vi "Poke-n-probe.vi"(6 "Tries":i32=150, 7 "Goal":T1, 8 "error in":errorcluster, 9 "Speed":dbl=15.0, 10 "Zone":dbl=5.0, 11 "Location":string="Base") -> (0 "error out":errorcluster, 1 "Speed Out":dbl, 2 "Success":bool, 3 "Location Out":string="Base", 5 "Pose":T1)   [LabVIEW 2013]
uses:
  ROS/Code/Console/Servers/ServerSubs/(nist) Arm Globals.vi
panel:
  in  "Tolerance":dbl
  out "Overload":dbl
  out "Try":i32
  in  "stop":bool
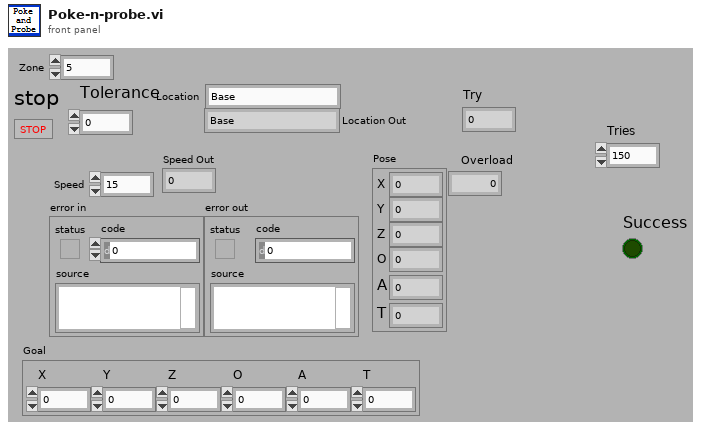
[diagram p1: front panel]
types:
  T1 = cluster{"X":dbl, "Y":dbl, "Z":dbl, "O":dbl, "A":dbl, "T":dbl}
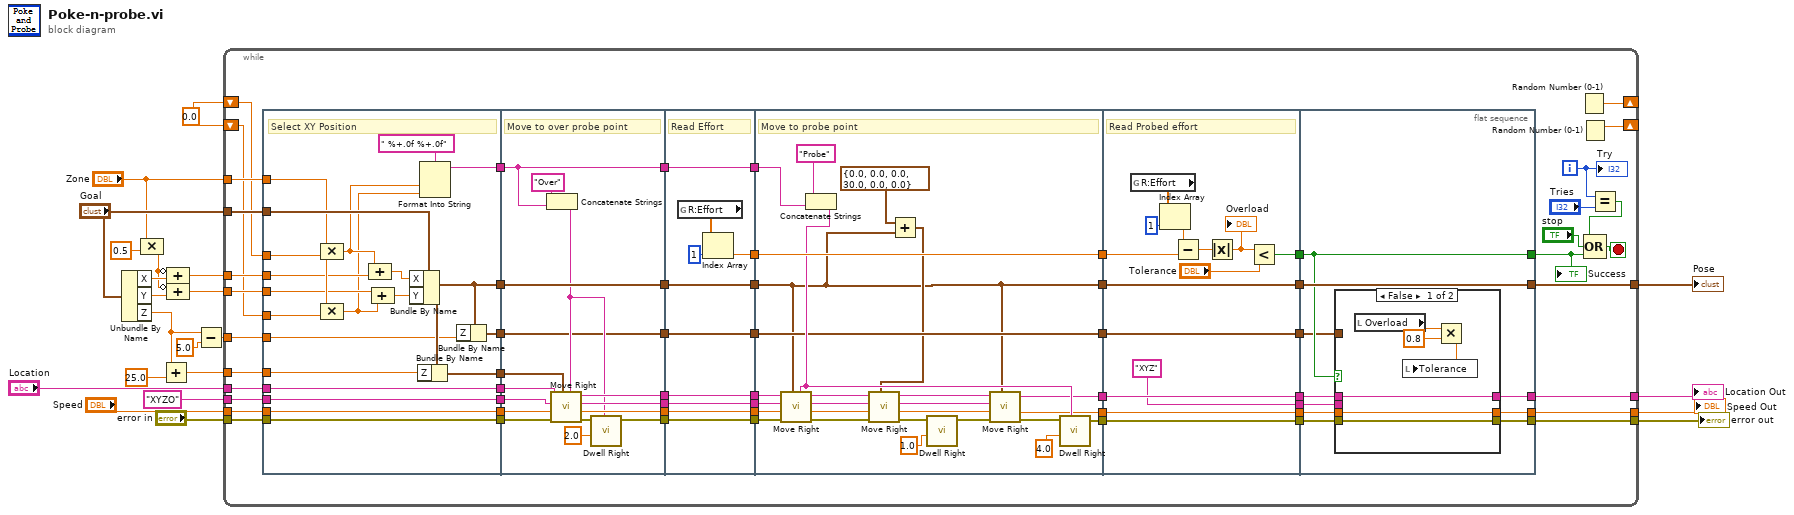
[diagram p0: block diagram]
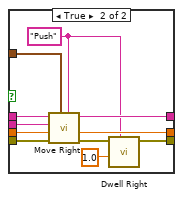
[diagram p2: hidden frame]
diagram:
  w1 = 0.0
  n1 = Unbundle By Name("Goal") -> ("X"=w15:dbl, "Y"=w14:dbl, "Z"=w4:dbl)
  n2 = Compound Arithmetic op=MULTIPLY("Zone", 0.5 ("value")) -> (w12:dbl)
  n3 = Add(x=w4, y=25.0 ("x")) -> (x+y=w17:dbl)
  n4 = Compound Arithmetic op=ADD(invert w12, w15) -> (w9:dbl)
  n5 = Compound Arithmetic op=ADD(invert w12, w14) -> (w10:dbl)
  n6 = Subtract(x=w4, y=5.0) -> (x-y=w2:dbl)
  n7 = while {
    tunnel: "error in" -> [w64]
    tunnel: "Location" -> [w63]
    tunnel: "XYZO" ("Mask") -> [w62]
    tunnel: "Speed" -> [w61]
    tunnel: w17 -> [w60]
    tunnel: "Goal" -> [w59]
    tunnel: "Zone" -> [w58]
    tunnel: w10 -> [w57]
    tunnel: w9 -> [w56]
    tunnel: [w54] -> w8
    tunnel: [w53] -> w5
    tunnel: [w51] -> w7
    tunnel: [w50] -> w6
    tunnel: w2 -> [w34]
    shift-right: [w24] -> _
    shift-left: w1 -> [w26]
    shift-right: [w23] -> _
    shift-left: w1 -> [w25]
    i -> [w42]
    stop <- w48 stop-if-true
    n8 = flat-sequence {
      tunnel: w61 -> [w100]
      tunnel: w62 -> [w101]
      tunnel: w63 -> [w102]
      tunnel: w64 -> [w103]
      tunnel: [w103] -> w82
      tunnel: [w102] -> w81
      tunnel: [w101] -> w80
      tunnel: [w100] -> w79
      tunnel: w60 -> [w99]
      tunnel: [w98] -> w78
      tunnel: [w87] -> w77
      tunnel: w59 -> [w97]
      tunnel: w58 -> [w96]
      tunnel: w57 -> [w95]
      tunnel: w56 -> [w94]
      tunnel: [w90] -> w46
      tunnel: w34 -> [w86]
      tunnel: [w85] -> w29
      tunnel: w26 -> [w84]
      tunnel: w25 -> [w83]
      tunnel: w82 -> [w119]
      tunnel: w81 -> [w118]
      tunnel: w80 -> [w116]
      tunnel: w79 -> [w115]
      tunnel: w78 -> [w117]
      tunnel: w77 -> [w113]
      tunnel: [w113] -> w76
      tunnel: [w112] -> w75
      tunnel: [w111] -> w74
      tunnel: [w110] -> w73
      tunnel: [w109] -> w72
      tunnel: w46 -> [w106]
      tunnel: [w106] -> w44
      tunnel: [w104] -> w30
      tunnel: w29 -> [w104]
      tunnel: [w127] -> w71
      tunnel: w76 -> [w127]
      tunnel: [w126] -> w70
      tunnel: w75 -> [w126]
      tunnel: [w125] -> w69
      tunnel: w74 -> [w125]
      tunnel: [w124] -> w68
      tunnel: w73 -> [w124]
      tunnel: [w123] -> w67
      tunnel: w72 -> [w123]
      tunnel: [w122] -> w66
      tunnel: [w121] -> w45
      tunnel: w44 -> [w121]
      tunnel: [w120] -> w31
      tunnel: w30 -> [w120]
      tunnel: w71 -> [w133]
      tunnel: w70 -> [w155]
      tunnel: w69 -> [w154]
      tunnel: w68 -> [w153]
      tunnel: w67 -> [w152]
      tunnel: [w151] -> w65
      tunnel: w66 -> [w151]
      tunnel: [w150] -> w55
      tunnel: [w133] -> w52
      tunnel: w45 -> [w148]
      tunnel: [w146] -> w32
      tunnel: w31 -> [w146]
      tunnel: [w134] -> w28
      tunnel: [w131] -> w27
      tunnel: w65 -> [w167]
      tunnel: w55 -> [w161]
      tunnel: w52 -> [w160]
      tunnel: [w165] -> w40
      tunnel: [w164] -> w39
      tunnel: [w162] -> w38
      tunnel: [w161] -> w37
      tunnel: [w160] -> w36
      tunnel: ["XYZ" ("Mask")] -> w35
      tunnel: [w159] -> w33
      tunnel: w32 -> [w159]
      tunnel: w28 -> [w164]
      tunnel: w27 -> [w165]
      tunnel: [w180] -> w53
      tunnel: [w175] -> w54
      tunnel: [w172] -> w49
      tunnel: [w173] -> w50
      tunnel: [w174] -> w51
      tunnel: w40 -> [w179]
      tunnel: w39 -> [w176]
      tunnel: w38 -> [w172]
      tunnel: w37 -> [w177]
      tunnel: w36 -> [w180]
      tunnel: w35 -> [w178]
      tunnel: w33 -> [w171]
      frame #0 {
        # "Select XY Position"
        n9 = Compound Arithmetic op=MULTIPLY(w96, w84) -> (w89:dbl)
        n10 = Compound Arithmetic op=MULTIPLY(w96, w83) -> (w88:dbl)
        n11 = Compound Arithmetic op=ADD(w89, w94) -> (w92:dbl)
        n12 = Compound Arithmetic op=ADD(w95, w88) -> (w91:dbl)
        n13 = Bundle By Name(cluster=w97, "X"=w92, "Y"=w91) -> (w87:T1)
        n14 = Bundle By Name(cluster=w87, "Z"=w99) -> (w98:T1)
        n15 = Format Into String(format string=" %+.0f %+.0f", w89, w88) -> (resulting string=w90:string)  [unwired: 2 in, 1 out]
        n16 = Bundle By Name(cluster=w87, "Z"=w86) -> (w85:T1)
      }
      frame #1 {
        # "Move to over probe point"
        n17 = Concatenate Strings("Over" ("string"), w106) -> (w105:string)
        n18 = call "Move Right.vi"("Label"=w105, "Goal"=w117, "error in"=w119, "Speed"=w115, "Mask"=w116, "Location"=w118) -> ("error out"=w114:errorcluster, "Speed Out"=w110:dbl, "Mask Out"=w111:string, "Location Out"=w112:string)  [unwired: 1 in, 1 out]
        n19 = call "Dwell Right.vi"("Label"=w105, "Wait Time"=2.0, "error in"=w114) -> ("error out"=w109:errorcluster)  [unwired: 8 in]
      }
      frame #2 {
        # "Read Effort"
        n20 = global read "(nist) Arm Globals.vi" "R:Effort"() -> (w129:dbl[])
        n21 = Index Array(array=w129, index=1) -> (element=w122:dbl)
      }
      frame #3 {
        # "Move to probe point"
        n22 = Concatenate Strings("Probe" ("Label"), w148) -> (w147:string)
        n23 = call "Move Right.vi"("Label"=w147, "Goal"=w133, "error in"=w152, "Speed"=w153, "Mask"=w154, "Location"=w155) -> ("error out"=w145:errorcluster, "Speed Out"=w144:dbl, "Mask Out"=w141:string, "Location Out"=w143:string)  [unwired: 1 in, 1 out]
        n24 = Add(x=T1 {"X"=0.0, "Y"=0.0, "Z"=0.0, "O"=30.0, "A"=0.0, "T"=0.0} ("y"), y=w133) -> (x+y=w142:T1)
        n25 = call "Move Right.vi"("Goal"=w142, "error in"=w145, "Speed"=w144, "Mask"=w141, "Location"=w143) -> ("error out"=w139:errorcluster, "Speed Out"=w135:dbl, "Mask Out"=w130:string, "Location Out"=w132:string)  [unwired: 2 in, 1 out]
        n26 = call "Dwell Right.vi"("Wait Time"=1.0, "error in"=w139) -> ("error out"=w137:errorcluster)  [unwired: 9 in]
        n27 = call "Move Right.vi"("Goal"=w133, "error in"=w137, "Speed"=w135, "Mask"=w130, "Location"=w132) -> ("error out"=w136:errorcluster, "Speed Out"=w134:dbl, "Location Out"=w131:string)  [unwired: 2 in, 2 out]
        n28 = call "Dwell Right.vi"("Label"=w147, "Wait Time"=4.0, "error in"=w136) -> ("error out"=w150:errorcluster)  [unwired: 8 in]
      }
      frame #4 {
        # "Read Probed effort"
        n29 = global read "(nist) Arm Globals.vi" "R:Effort"() -> (w170:dbl[])
        n30 = Index Array(array=w170, index=1) -> (element=w168:dbl)
        n31 = Subtract(x=w168, y=w167) -> (x-y=w166:dbl)
        n32 = Absolute Value(x=w166) -> (abs(x)=w163:dbl)
        "Overload" <- w163
        n33 = Less?(x=w163, y="Tolerance") -> (x < y?=w162:bool)
      }
      frame #5 {
        n34 = case shown="False" w172 {
          tunnel: w179 -> [w186 w195]
          tunnel: w178 -> [_ w194]
          tunnel: w177 -> [w184 w193]
          tunnel: w176 -> [w185 w192]
          tunnel: [w184 w191] -> w175
          tunnel: [w186 w190] -> w174
          tunnel: [w185 w189] -> w173
          tunnel: w171 -> [_ w187]
          frame False {
            n35 = local read "Overload"() -> (w183:dbl)
            n36 = Multiply(x=w183, y=0.8) -> (x*y=w182:dbl)
            n37 = local write "Tolerance"(w182) -> ()
          }
          frame True {
            w188 = "Push" ("Label")
            n38 = call "Move Right.vi"("Label"=w188, "Goal"=w187, "error in"=w193, "Speed"=w192, "Mask"=w194, "Location"=w195) -> ("error out"=w196:errorcluster, "Speed Out"=w189:dbl, "Location Out"=w190:string)  [unwired: 1 in, 2 out]
            n39 = call "Dwell Right.vi"("Label"=w188, "Wait Time"=1.0, "error in"=w196) -> ("error out"=w191:errorcluster)  [unwired: 8 in]
          }
        }
      }
    }
    n40 = Random Number (0-1)() -> (number: 0 to 1=w24:dbl)
    n41 = Random Number (0-1)() -> (number: 0 to 1=w23:dbl)
    n42 = Equal?(x=w42, y="Tries") -> (x = y?=w41:bool)
    n43 = Compound Arithmetic op=OR(w41, "stop", w49) -> (w48:bool)
    "Try" <- w42
    "Success" <- w49
  }
  "error out" <- w8
  "Location Out" <- w7
  "Speed Out" <- w6
  "Pose" <- w5
